vi "Read Test Value.vi"(8 "error in (no error)":errorcluster, 11 "Test in":refnum<class "Test.lvclass">) -> (0 "error out":errorcluster, 2 "Value":dbl, 3 "Test out":refnum<class "Test.lvclass">)   [LabVIEW 2014, in "Test.lvclass"]
uses:
  Test.lvclass
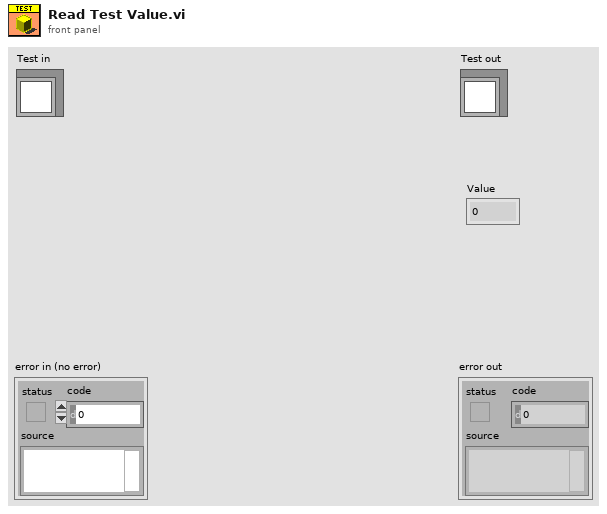
[diagram p1: front panel]
types:
  T1 = typedef "Test.lvclass/ObjectAttributes.ctl" = cluster{"Value":dbl}
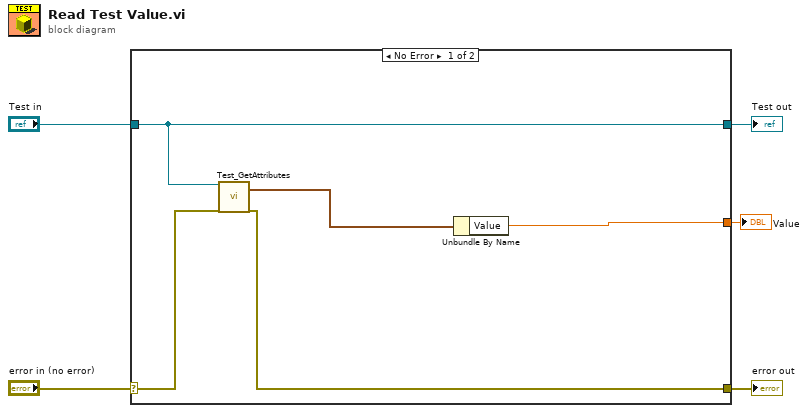
[diagram p0: block diagram]
diagram:
  n1 = case shown="No Error" "error in (no error)" {
    selector: "error in (no error)" -> [w9 w12]
    tunnel: [w6 w12] -> w4
    tunnel: [w10 w11] -> w2
    tunnel: "Test in" -> [w10 w11]
    tunnel: [w7 _] -> w1
    frame No Error {
      n2 = call "Test_GetAttributes.vi"("reference in"=w10, "error in (no error)"=w9) -> ("Data"=w8:T1, "error out"=w6:errorcluster)  [unwired: 14 in, 2 out]
      n3 = Unbundle By Name(w8) -> ("Value"=w7:dbl)
    }
    frame Error {
    }
  }
  "error out" <- w4
  "Test out" <- w2
  "Value" <- w1
